vi "1A Helper - Init Sensor.vi"(8 "error in (no error)":errorcluster, 11 "VISA Refnum in":refnum<visa-resource-name>="COM1") -> (0 "error out":errorcluster, 2 "Try #":i32, 3 "VISA Refnum out":refnum<visa-resource-name>)   [LabVIEW 2011]
doc: "This VI checks to see if the sensor is communicating on 4800 or 38400 baud and sets it to 38400 baud if it is not already."
uses:
  2-Think/2 Typedefs/indicator LED.ctl
  2-Think/2 Globals/2 Global.vi
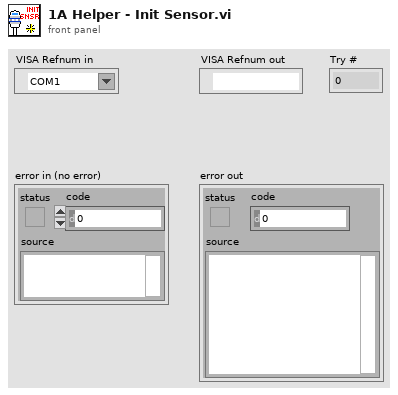
[diagram p1: front panel]
types:
  T1 = typedef "indicator LED.ctl" = bool
  T2 = typedef "generalized sensor status.ctl" = cluster{"Sensor Connected":T1, "Sensor Initialized":T1, "Sensor OK":T1, "Latest Error String":string, "GPS Lock":T1}
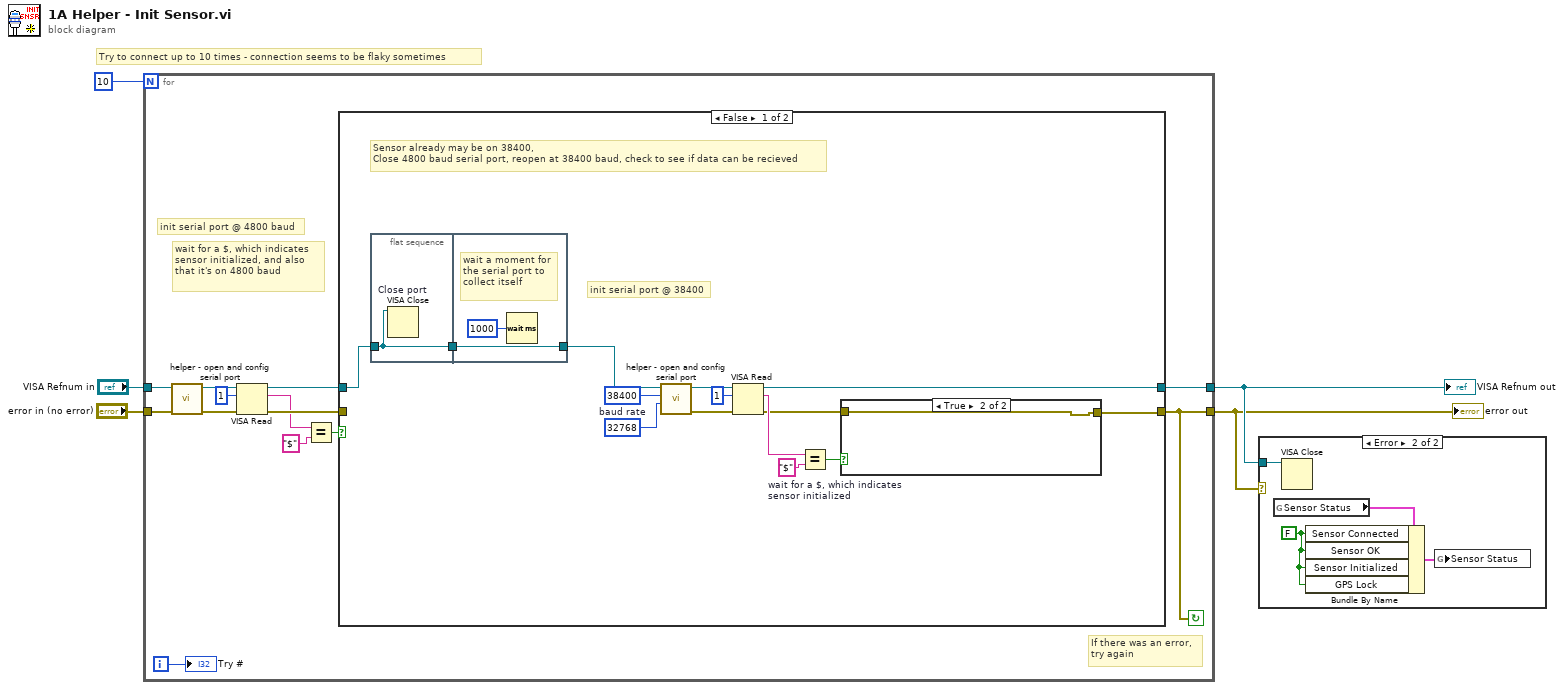
[diagram p0: block diagram]
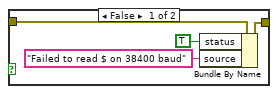
[diagram p2: hidden frame]
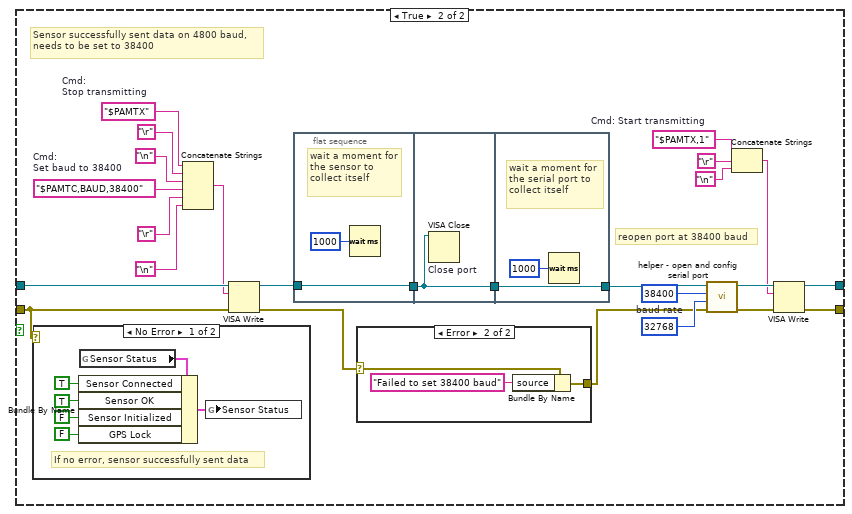
[diagram p3: hidden frame]
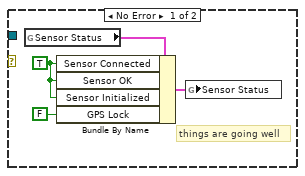
[diagram p6: hidden frame]
diagram:
  # "Try to connect up to 10 times - connection seems to be flaky sometimes"
  n1 = for {
    N: 10 -> [_]
    tunnel: "error in (no error)" -> [w18]
    tunnel: "VISA Refnum in" -> [w17]
    tunnel: [w16] -> w3
    tunnel: [w7] -> w2
    i -> [w6]
    stop <- w7 continue-if-true
    # "If there was an error, \ntry again"
    # "wait for a $, which indicates sensor initialized, and also that it's on 4800 baud"
    # "init serial port @ 4800 baud"
    n2 = call "helper - open and config serial port.vi"("error in (no error)"=w18, "VISA Refnum in"=w17) -> ("error out"=w13:errorcluster, "VISA Refnum out"=w14:refnum<visa-resource-name>)  [unwired: 8 in]
    n3 = VISA Read(VISA resource name=w14, byte count=u32 1, error in (no error)=w13) -> (VISA resource name out=w15:refnum<visa-resource-name>, read buffer=w9:string, error out=w12:errorcluster)  [unwired: 1 out]
    n4 = Equal? ("wait for a $, which indicates\nsensor initialized")(x=w9, y="$" ("x")) -> (x = y?=w11:bool)
    n5 = case shown="False" w11 {
      tunnel: [w28 w61] -> w16
      tunnel: w15 -> [w25 w53]
      tunnel: w12 -> [_ w43]
      tunnel: [w27 w48] -> w7
      frame False {
        w32 = u32 38400  # baud rate
        # "init serial port @ 38400"
        # "Sensor already may be on 38400,\nClose 4800 baud serial port, reopen at 38400 baud, check to see if data can be recieved"
        n6 = flat-sequence {
          tunnel: [w38] -> w26
          tunnel: w25 -> [w38]
          tunnel: [w40] -> w24
          tunnel: w26 -> [w40]
          frame #0 {
            n7 = VISA Close "Close port"(VISA resource name=w38) -> ()  [unwired: 1 in, 1 out]
          }
          frame #1 {
            # "wait a moment for the serial port to collect itself"
            n8 = Wait (ms)(milliseconds to wait=u32 1000) -> ()  [unwired: 1 out]
          }
        }
        n9 = call "helper - open and config serial port.vi"("Input\nbuffer size"=u32 32768 ("Input\nbuffer size"), "baud rate"=w32, "VISA Refnum in"=w24) -> ("error out"=w29:errorcluster, "VISA Refnum out"=w30:refnum<visa-resource-name>)  [unwired: 7 in]
        n10 = VISA Read(VISA resource name=w30, byte count=u32 1, error in (no error)=w29) -> (VISA resource name out=w28:refnum<visa-resource-name>, read buffer=w22:string, error out=w19:errorcluster)  [unwired: 1 out]
        n11 = Equal? "wait for a $, which indicates\nsensor initialized"(x=w22, y="$" ("x")) -> (x = y?=w20:bool)
        n12 = case shown="True" w20 {
          tunnel: w19 -> [w34 w37]
          tunnel: [w33 w37] -> w27
          frame False {
            n13 = Bundle By Name(cluster=w34, "status"=TRUE, "source"="Failed to read $ on 38400 baud") -> (w33:errorcluster)
          }
          frame True {
          }
        }
      }
      frame True {
        w47 = "$PAMTC,BAUD,38400"  # Cmd: Set baud to 38400
        w52 = "$PAMTX"  # Cmd: Stop transmitting
        w57 = "$PAMTX,1"  # Cmd: Start transmitting
        w63 = u32 38400  # baud rate
        # "Sensor successfully sent data on 4800 baud,\nneeds to be set to 38400"
        # "reopen port at 38400 baud"
        n14 = case shown="No Error" w43 {
          frame No Error {
            # "If no error, sensor successfully sent data"
            n15 = global read "2 Global.vi" "Sensor Status"() -> (w74:T2)
            n16 = Bundle By Name(cluster=w74, "Sensor Connected"=T1 TRUE, "Sensor OK"=T1 TRUE, "Sensor Initialized"=T1 FALSE, "GPS Lock"=T1 FALSE) -> (w75:T2)
            n17 = global write "2 Global.vi" "Sensor Status"(w75) -> ()
          }
          frame Error {
          }
        }
        n18 = Concatenate Strings(w52, "\r" ("Carriage Return Constant"), "\n", w47, "\r" ("Carriage Return Constant"), "\n") -> (w51:string)
        n19 = VISA Write(VISA resource name=w53, write buffer=w51, error in (no error)=w43) -> (VISA resource name out=w44:refnum<visa-resource-name>, error out=w42:errorcluster)  [unwired: 1 out]
        n20 = flat-sequence {
          tunnel: w44 -> [w76]
          tunnel: [w76] -> w65
          tunnel: w65 -> [w78]
          tunnel: [w78] -> w64
          tunnel: [w80] -> w62
          tunnel: w64 -> [w80]
          frame #0 {
            # "wait a moment for the sensor to collect itself"
            n21 = Wait (ms)(milliseconds to wait=u32 1000) -> ()  [unwired: 1 out]
          }
          frame #1 {
            n22 = VISA Close "Close port"(VISA resource name=w78) -> ()  [unwired: 1 in, 1 out]
          }
          frame #2 {
            # "wait a moment for the serial port to collect itself"
            n23 = Wait (ms)(milliseconds to wait=u32 1000) -> ()  [unwired: 1 out]
          }
        }
        n24 = case shown="Error" w42 {
          selector: w42 -> [w66 w69]
          tunnel: [w66 w67] -> w41
          frame No Error {
          }
          frame Error {
            n25 = Bundle By Name(cluster=w69, "source"="Failed to set 38400 baud") -> (w67:errorcluster)
          }
        }
        n26 = call "helper - open and config serial port.vi"("error in (no error)"=w41, "Input\nbuffer size"=u32 32768 ("Input\nbuffer size"), "baud rate"=w63, "VISA Refnum in"=w62) -> ("error out"=w60:errorcluster, "VISA Refnum out"=w58:refnum<visa-resource-name>)  [unwired: 6 in]
        n27 = Concatenate Strings(w57, "\r" ("Carriage Return Constant"), "\n") -> (w54:string)
        n28 = VISA Write(VISA resource name=w58, write buffer=w54, error in (no error)=w60) -> (VISA resource name out=w61:refnum<visa-resource-name>, error out=w48:errorcluster)  [unwired: 1 out]
      }
    }
    "Try #" <- w6
  }
  "VISA Refnum out" <- w3
  "error out" <- w2
  n29 = case shown="Error" w2 {
    tunnel: w3 -> [_ w88]
    frame No Error {
      w82 = T1 TRUE ("Sensor Connected")
      # "things are going well"
      n30 = global read "2 Global.vi" "Sensor Status"() -> (w83:T2)
      n31 = Bundle By Name(cluster=w83, "Sensor Connected"=w82, "Sensor OK"=w82, "Sensor Initialized"=w82, "GPS Lock"=T1 FALSE) -> (w84:T2)
      n32 = global write "2 Global.vi" "Sensor Status"(w84) -> ()
    }
    frame Error {
      w85 = T1 FALSE ("Sensor Connected")
      n33 = global read "2 Global.vi" "Sensor Status"() -> (w86:T2)
      n34 = VISA Close(VISA resource name=w88) -> ()  [unwired: 1 in, 1 out]
      n35 = Bundle By Name(cluster=w86, "Sensor Connected"=w85, "Sensor OK"=w85, "Sensor Initialized"=w85, "GPS Lock"=w85) -> (w87:T2)
      n36 = global write "2 Global.vi" "Sensor Status"(w87) -> ()
    }
  }
